vi "Inverse f Designer.vi"(5 "fs":dbl=1.0 format="%.2f", 6 "order":i32=5, 7 "exponent":dbl=1.0 format="%.2g", 8 "higher cutoff freq":dbl=0.5, 9 "lower cutoff freq":dbl=0.1) -> (0 "error":i32, 1 "b[i]":dbl[](array[numeric]) format="%.2f", 3 "a[i]":dbl[](array[numeric]) format="%.2f", 4 "fmin":dbl=1.5811388300841898e-05 format="%.2f")   [LabVIEW 2017, in "NI_AALBase.lvlib"]
doc: "This VI designs a 1/f filter covering the frequency range defined by lower and higher cutoff frequencies. order sets the total number of 1st order stages to be designed.\n\nexponent is the negative exponent of the desired magnitude-squared response ( |S(f)| = 1/f^exponent ).\n\nThe formulas for each real zero and pole for the 1st order stages are (from highest to lowest frequency):\nfor i = 0 .. N-1\n zi = exp(-2PI fzi)\n pi = exp(-2PI fpi)\nwhere\n fzi = fmax * 10^(-i/h)\n fpi = fzi * 10^(-g/(2*h))\n\nGiven the equation for each stage:\n y(n) = x(n) + bx(n-1) - ay(n-1)\n\nThe coefficients ai and bi are:\n ai = -zi = -exp(-2PI fpi)\n bi = -pi = -exp(-2PI fzi)\n\nReference\n---------\nCorsini and Saletti, \"A 1/f^ Power Spectrum Noise Sequence Generator\", IEEE Transactions on Instrumentation and Measurement, Vol 37, No.4, Dec 1988"
uses:
  <vilib>/Analysis/NI_AALBase.lvlib
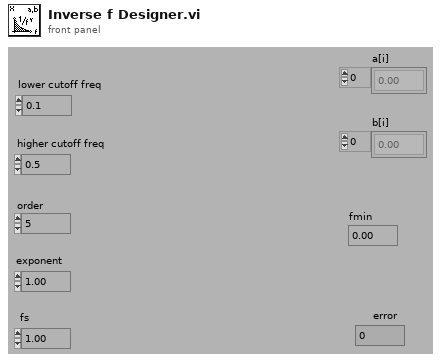
[diagram p1: front panel]
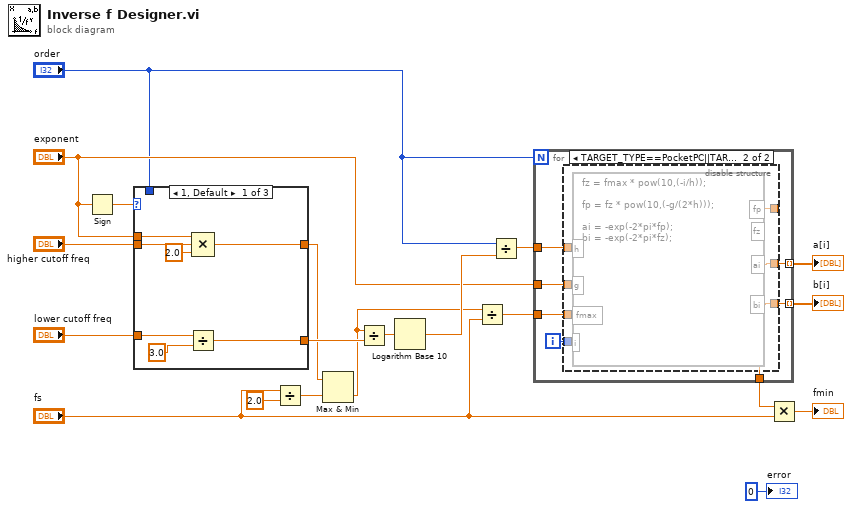
[diagram p0: block diagram]
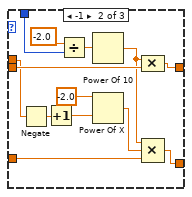
[diagram p2: hidden frame]
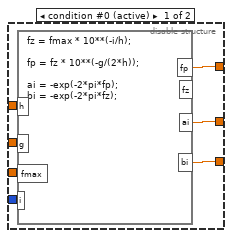
[diagram p4: hidden frame]
diagram:
  n1 = Sign(1:"exponent") -> (0:w4:dbl)
  n2 = case shown="1, Default" w4 {
    tunnel: "lower cutoff freq" -> [w27 w40 w41]
    tunnel: [w26 w39 w41] -> w10
    tunnel: "higher cutoff freq" -> [w25 w38 w42]
    tunnel: "exponent" -> [w23 w33 _]
    tunnel: [w21 w37 w42] -> w2
    tunnel: "order" -> [_ w28 _]
    frame 1, Default {
      n3 = Divide(x=w27, y=3.0) -> (x/y=w26:dbl)
      n4 = Compound Arithmetic op=MULTIPLY(w23, w25, 2.0 ("value")) -> (w21:dbl)
    }
    frame -1 {
      n5 = Negate(x=w33) -> (-x=w35:dbl)
      n6 = Increment(x=w35) -> (x+1=w34:dbl)
      n7 = Divide(x=-2.0, y=w28) -> (x/y=w31:dbl)
      n8 = Power Of 10(x=w31) -> (10^x=w29:dbl)
      n9 = Power Of X(1:w34, 2:-2.0 ("y")) -> (0:w30:dbl)
      n10 = Compound Arithmetic op=MULTIPLY(w29, w38) -> (w37:dbl)
      n11 = Compound Arithmetic op=MULTIPLY(w29, w30, w40) -> (w39:dbl)
    }
    frame 0 {
    }
  }
  n12 = Divide(x="fs", y=2.0) -> (x/y=w6:dbl)
  n13 = Max & Min(x=w2, y=w6) -> (min(x,y)=w5:dbl)  [unwired: 1 out]
  n14 = Divide(x=w5, y=w10) -> (x/y=w14:dbl)
  n15 = Logarithm Base 10(1:w14) -> (0:w13:dbl)
  n16 = Divide(x=w5, y="fs") -> (x/y=w16:dbl)
  n17 = Divide(x="order", y=w13) -> (x/y=w12:dbl)
  n18 = for {
    N: "order" -> [_]
    tunnel: w12 -> [w49]
    tunnel: "exponent" -> [w48]
    tunnel: w16 -> [w47]
    tunnel: [w45] -> w19 mode=indexing
    tunnel: [w44] -> w18 mode=indexing
    tunnel: [w43] -> w17
    i -> [w46]
    n19 = disable-structure shown="TARGET_TYPE==PocketPC||TARGET_TYPE==PalmOS||TARGET_TYPE==Embedded" {
      disable-tunnel: w49 -> [w56 w63]
      disable-tunnel: w48 -> [w55 w62]
      disable-tunnel: w47 -> [w54 w61]
      disable-tunnel: w46 -> [w53 w60]
      disable-tunnel: [w52 w59] -> w45
      disable-tunnel: [w51 w58] -> w44
      disable-tunnel: [w50 w57] -> w43
      frame condition #0 (active) {
        n20 = formula code="fz = fmax * 10**(-i/h);\n\nfp = fz * 10**(-g/(2*h));\n\nai = -exp(-2*pi*fp);\nbi = -exp(-2*pi*fz);"("h"=w56, "g"=w55, "fmax"=w54, "i"=w53) -> ("fp"=w50:dbl, "ai"=w52:dbl, "bi"=w51:dbl)  [unwired: 1 out]
      }
      frame condition #1 {
        n21 = formula code="fz = fmax * pow(10,(-i/h));\n\nfp = fz * pow(10,(-g/(2*h)));\n\nai = -exp(-2*pi*fp);\nbi = -exp(-2*pi*fz);"("h"=w63, "g"=w62, "fmax"=w61, "i"=w60) -> ("fp"=w57:dbl, "ai"=w59:dbl, "bi"=w58:dbl)  [unwired: 1 out]
      }
    }
  }
  "b[i]" <- w18
  "a[i]" <- w19
  n22 = Multiply(x=w17, y="fs") -> (x*y=→"fmin":dbl)
  "error" <- 0 ("error")
